vi "Large Single Write.vi"(5 "Username":string, 6 "Password":string, 7 "Address":string, 8 "Error In":errorcluster) -> (0 "Error Out":errorcluster)   [LabVIEW 2018, in "Tests.lvlib" / "SFTP File.lvlib"]
doc: "Note, by \"large\" we mean a file larger than the SFTP/SSH write packet size maximum of 30Kb."
uses:
  SFTP File.lvlib
  src/Toolkit/SFTP File/API/Typedefs/Flags.ctl
  src/Toolkit/Type Definitions/Permissions.ctl
  src/Toolkit/Type Definitions/Modes.ctl
  src/Toolkit/SFTP File/SFTP File.lvclass
  src/Toolkit/Toolkit.lvlib
  <vilib>/addons/_JKI Toolkits/Caraya/classes/Test/Test.lvclass
  <vilib>/addons/_JKI Toolkits/Caraya/classes/Assert/Assert.lvclass
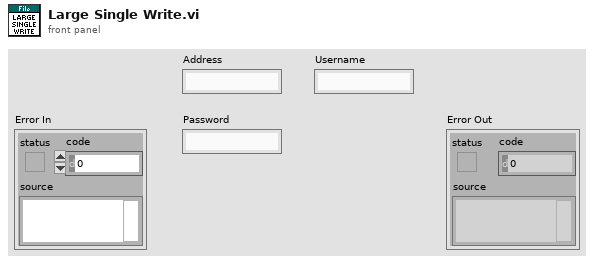
[diagram p1: front panel]
types:
  T1 = enum16{"open", "replace", "create", "open or create", "replace or create", "replace or create with confirmation"}
  T2 = typedef "Toolkit.lvlib/Permissions.ctl" = cluster{"Owner":T3, "Group":T3, "Others":T3}
  T3 = typedef "Toolkit.lvlib/Modes.ctl" = cluster{"Read":bool, "Write":bool, "Execute":bool}
  T4 = typedef "Toolkit.lvlib/SFTP File.lvclass/Flags.ctl" = cluster{"Read":bool, "Write":bool, "Append":bool, "Create":bool, "Truncate":bool, "Exclude":bool}
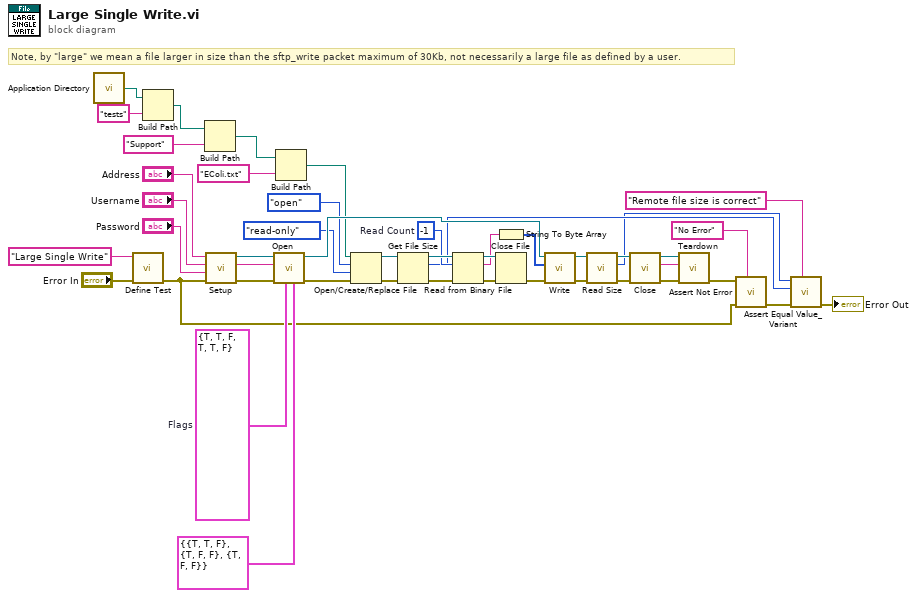
[diagram p0: block diagram]
diagram:
  w21 = -1  # Read Count
  w41 = T4 {"Read"=TRUE, "Write"=TRUE, "Append"=FALSE, "Create"=TRUE, "Truncate"=TRUE, "Exclude"=FALSE}  # Flags
  # "Note, by \"large\" we mean a file larger in size than the sftp_write packet maximum of 30Kb, not necessarily a large file as defined by a user."
  n1 = call <vilib>:"Application Directory.vi"() -> ("Application Directory"=w28:path)
  n2 = call <vilib>:"Define Test.vi"("error in (no error)"="Error In", "Label (VI Title)"="Large Single Write") -> ("error out"=w11:errorcluster)  [unwired: 9 in]
  n3 = Build Path(base path=w28, name or relative path="tests") -> (appended path=w26:path)
  n4 = Build Path(base path=w26, name or relative path="Support") -> (appended path=w24:path)
  n5 = call "Setup.vi"("Error In"=w11, "Password"="Password", "Username"="Username", "Address"="Address") -> ("Error Out"=w40:errorcluster, "Temporary File"=w29:string, "SFTP"=w43:refnum<class "SFTP.lvclass">)  [unwired: 5 in]
  n6 = call "Open.vi"("Permissions"=T2 {"Owner"={"Read"=TRUE, "Write"=TRUE, "Execute"=FALSE}, "Group"={"Read"=TRUE, "Write"=FALSE, "Execute"=FALSE}, "Others"={"Read"=TRUE, "Write"=FALSE, "Execute"=FALSE}}, "Flags"=w41, "Error In"=w40, "Remote Path"=w29, "SFTP"=w43) -> ("Error Out"=w35:errorcluster, "SFTP File"=w42:refnum<class "SFTP File.lvclass">)  [unwired: 5 in]
  n7 = Build Path(base path=w24, name or relative path="EColi.txt") -> (appended path=w23:path)
  n8 = Open/Create/Replace File(file path (use dialog)=w23, error in=w35, operation (0:open)=T1."open", access (0:read/write)=enum16{"read/write", "read-only", "write-only"}."read-only") -> (refnum out=w32:refnum<file>, error out=w30:errorcluster)  [unwired: 2 in, 1 out]
  n9 = Get File Size(file=w32, error in=w30) -> (refnum out=w31:refnum<file>, size (in bytes)=w6:i64, 0:w22:errorcluster)
  n10 = Read from Binary File(8:w22, 10:w21, 11:w31) -> (0:w17:errorcluster, 2:w19:string, 3:w20:refnum<file>)  [unwired: 3 in, 1 out]
  n11 = String To Byte Array(string=w19) -> (unsigned byte array=w18:u8[])
  n12 = Close File(refnum=w20, error in=w17) -> (error out=w16:errorcluster)  [unwired: 1 out]
  n13 = call "Write.vi"("Error In"=w16, "Data"=w18, "SFTP File In"=w42) -> ("Error Out"=w2:errorcluster, "SFTP File Out"=w5:refnum<class "SFTP File.lvclass">)  [unwired: 6 in, 1 out]
  n14 = call "Read Size.vi"("Error In"=w2, "SFTP File In"=w5) -> ("Error Out"=w3:errorcluster, "File Size"=w1:u64, "SFTP File Out"=w4:refnum<class "SFTP File.lvclass">)  [unwired: 7 in]
  n15 = call "Close.vi"("Error In"=w3, "SFTP File"=w4) -> ("Error Out"=w37:errorcluster, "Remote Path"=w39:string, "SFTP"=w38:refnum<class "SFTP.lvclass">)  [unwired: 7 in]
  n16 = call "Teardown.vi"("Error In"=w37, "Temporary File"=w39, "SFTP"=w38) -> ("Error Out"=w12:errorcluster)  [unwired: 8 in]
  n17 = call <vilib>:"Assert Not Error.vi"("Label"="No Error", "error in (no error)"=w11, "Not Error?"=w12) -> ("error out"=w9:errorcluster)  [unwired: 8 in]
  n18 = call <vilib>:"Assert Equal Value_Variant.vi"("Label"="Remote file size is correct", "error in (no error)"=w9, "Y"=w6, "X"=w1) -> ("error out"=→"Error Out":errorcluster)  [unwired: 7 in]
